vi "R45.vi"() -> ()   [LabVIEW 2016, in "beamline sections.lvlib"]
uses:
  controls/beamline sections.lvlib
  save load/saveloadprev.ctl
  <vilib>/Instr/_visa.llb/VISA Open Access Mode.ctl
  sub-VIs/sub-VIs.lvlib
  save load/SaveLoad.lvlib
panel:
  in  "Tab Control":T1(tab)
  out "ExB 2":bool
  in  "GFM Field set":dbl(slide) min=0.0 max=150.0 scale=0.0..2.0
  in  "ExB #2 Electric":dbl(slide) min=0.0 max=200.0 scale=0.0..60.0
  in  "Reset ExB 2":bool
  in  "ExB #1 Electric":dbl(slide) min=0.0 max=200.0 scale=0.0..60.0
  out "R45 Steerer Y Read":dbl format="%#.2g"
  out "R45 Steerer X Read":dbl format="%#.2g"
  in  "R45 Y steerer":dbl(slide) min=-10.0 max=10.0 scale=-10.0..10.0
  in  "R45 Quad A":dbl(slide) min=0.0 max=200.0 scale=0.0..120.0
  in  "R45 X steerer":dbl(slide) min=-10.0 max=10.0 scale=-10.0..10.0
  out "R45 Steerer":bool
  out "R45 quad Range":bool
  in  "R45 Quad B":dbl(slide) min=0.0 max=200.0 scale=0.0..120.0
  in  "stop":bool
  out "ExB 1":bool
  out "ExB 1- V":dbl format="%#.2g"
  in  "ExB #1 Magnet":dbl(slide) scale=0.0..30.0
  out "ExB 1+ V":dbl format="%#.2g"
  out "read current quad B":string
  out "read voltage quad B":string
  out "read current quad A":string
  out "read voltage Quad A":string
  in  "ExB #2 Magnet":dbl(slide) scale=0.0..30.0
  in  "Preview-Save-Load":T2
  out "ExB 2+ I":dbl
  out "ExB 2- I":dbl
  out "ExB 2- V":dbl
  out "ExB 2+ V":dbl
  out "ExB 1+ I":dbl
  out "ExB 1- I":dbl
  out "GFM field read":dbl
  out "Left-Steerer V read":dbl
  out "Down-Steerer V read":dbl
  out "Up-Steerer V read":dbl
  out "Right-Steerer V read":dbl
  out "Left-Steerer I read":dbl
  out "Right-Steerer I read":dbl
  out "Down-Steerer I read":dbl
  out "Up-Steerer I read":dbl
  in  "R45 temp file":path=path "D:/Main Tune Parameters/Temp Configs/R45.txt"
  in  "Quad A VISA GPIB Resource":refnum<visa-resource-name>="GPIB1::6::INSTR"
  in  "Quad B VISA GPIB Resource":refnum<visa-resource-name>="GPIB1::3::INSTR"
  out "SV error":errorcluster
  out "Quad B error":errorcluster
  out "Quad A error":errorcluster
  out "GFM SV error":errorcluster
  out "SaveLoad error":errorcluster
  out "R45-2-RT Error":errorcluster
  out "R45-2-FPGA Error":errorcluster
  out "R45-1-RT Error":errorcluster
  out "R45-1-FPGA Error":errorcluster
  # "R45"
  # "R45 X and Y steerers are split between Up/Down (Y) and Right/Left (X)"
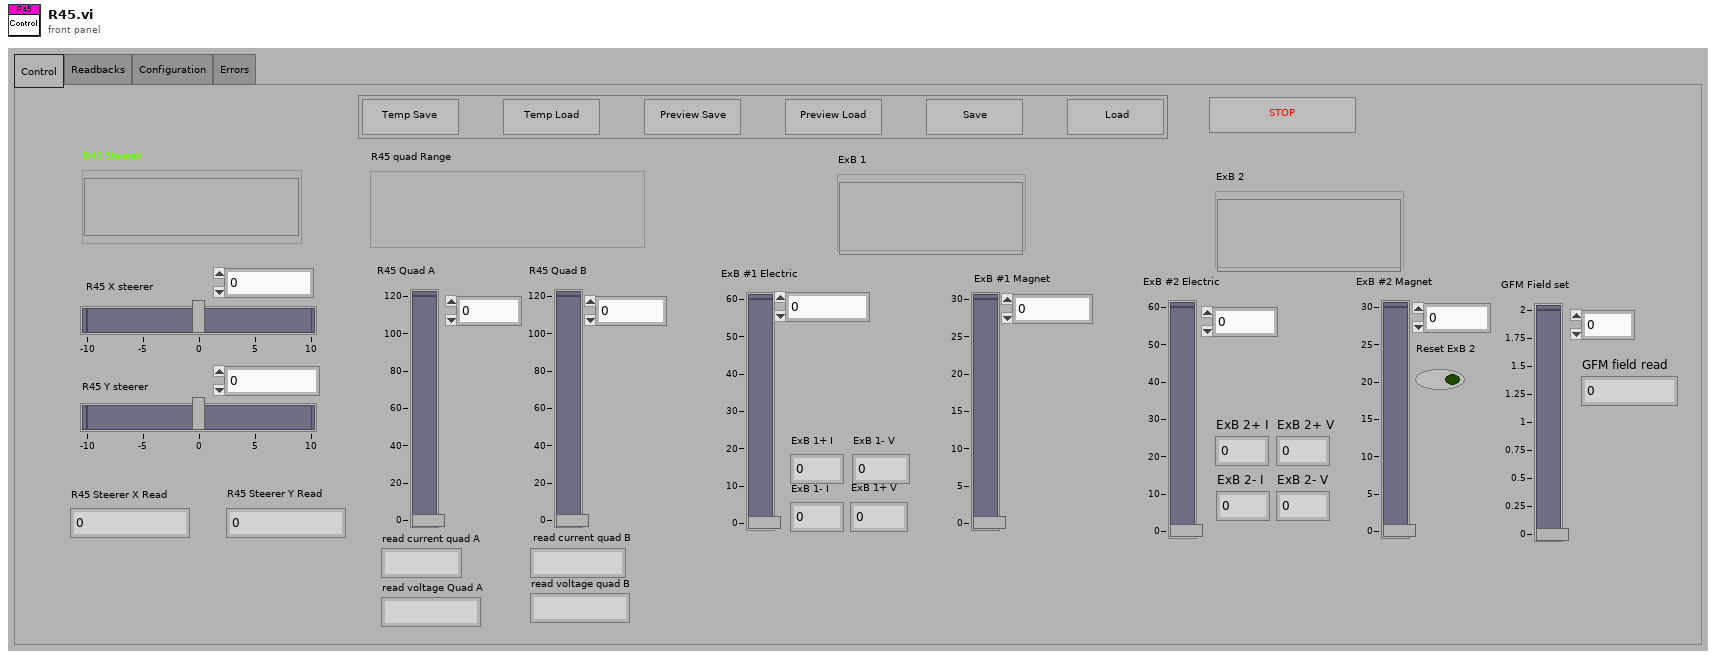
[diagram p1: front panel]
types:
  T1 = enum32{"Control", "Readbacks", "Configuration", "Errors"}
  T2 = typedef "saveloadprev.ctl" = cluster{"Temp Save":bool, "Temp Load":bool, "Save":bool, "Load":bool, "Preview Save":bool, "Preview Load":bool}
  T3 = typedef "VISA Open Access Mode.ctl" = u32
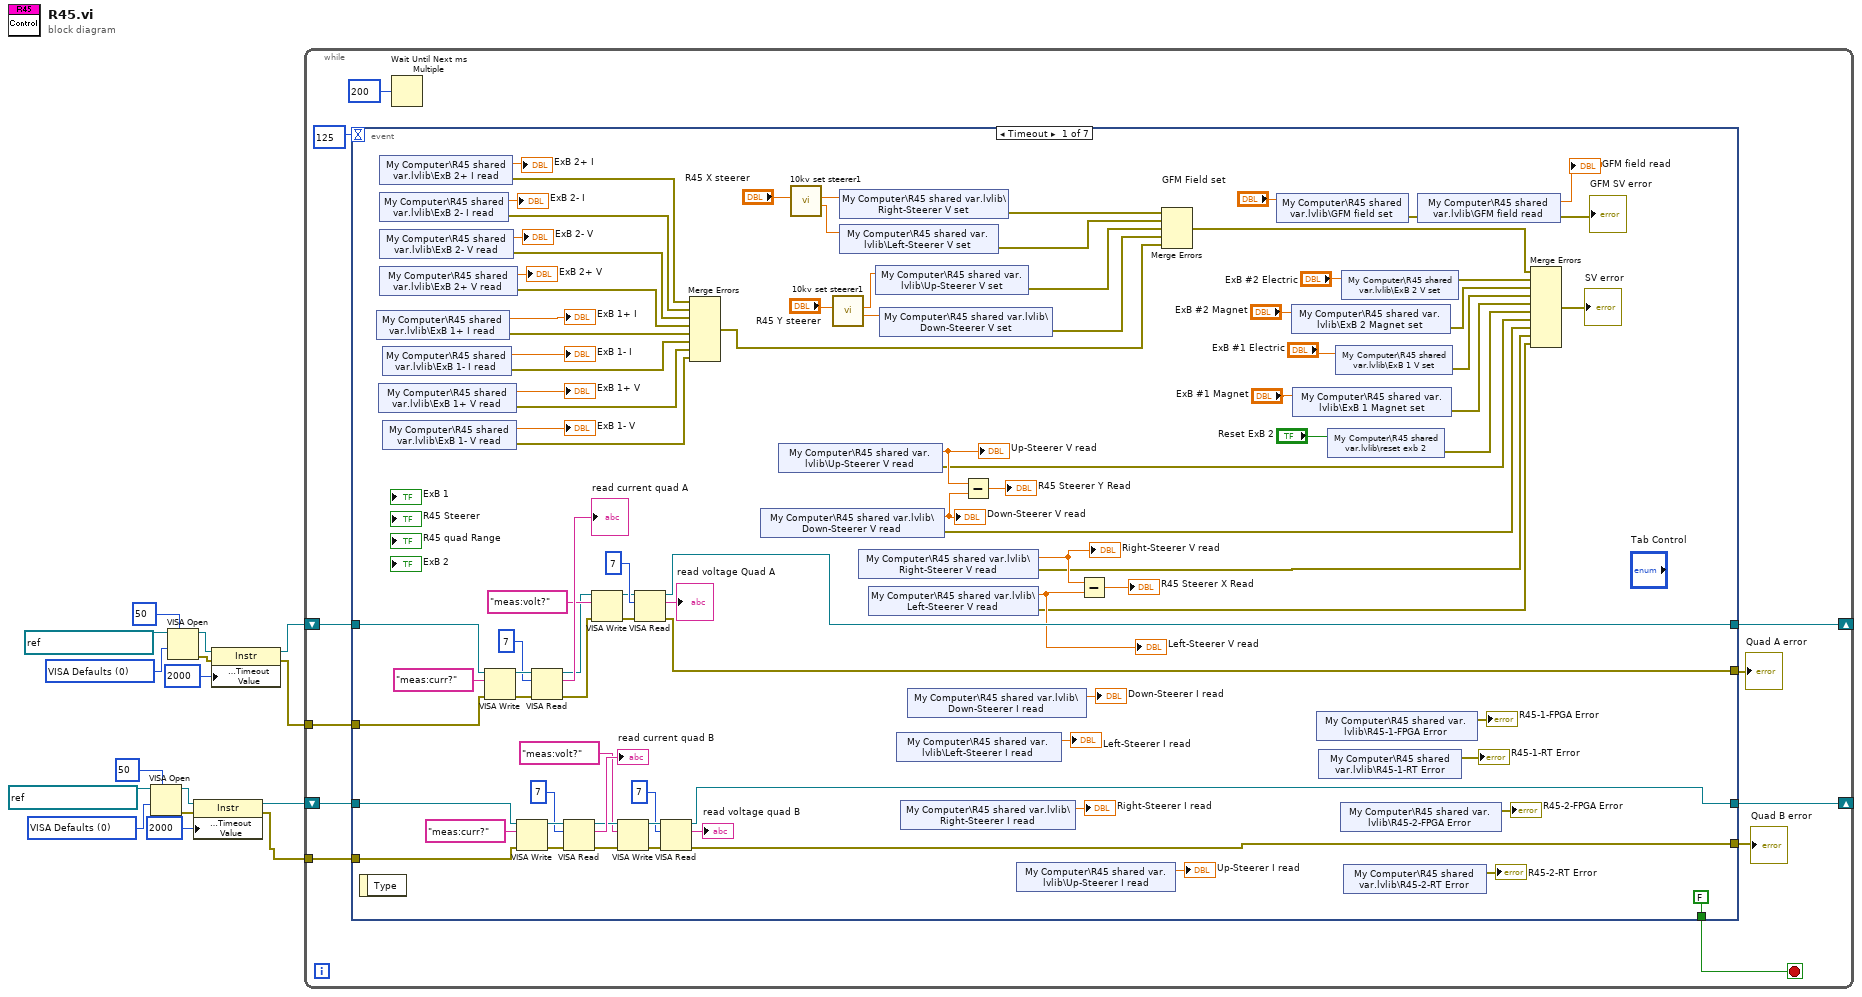
[diagram p0: block diagram]
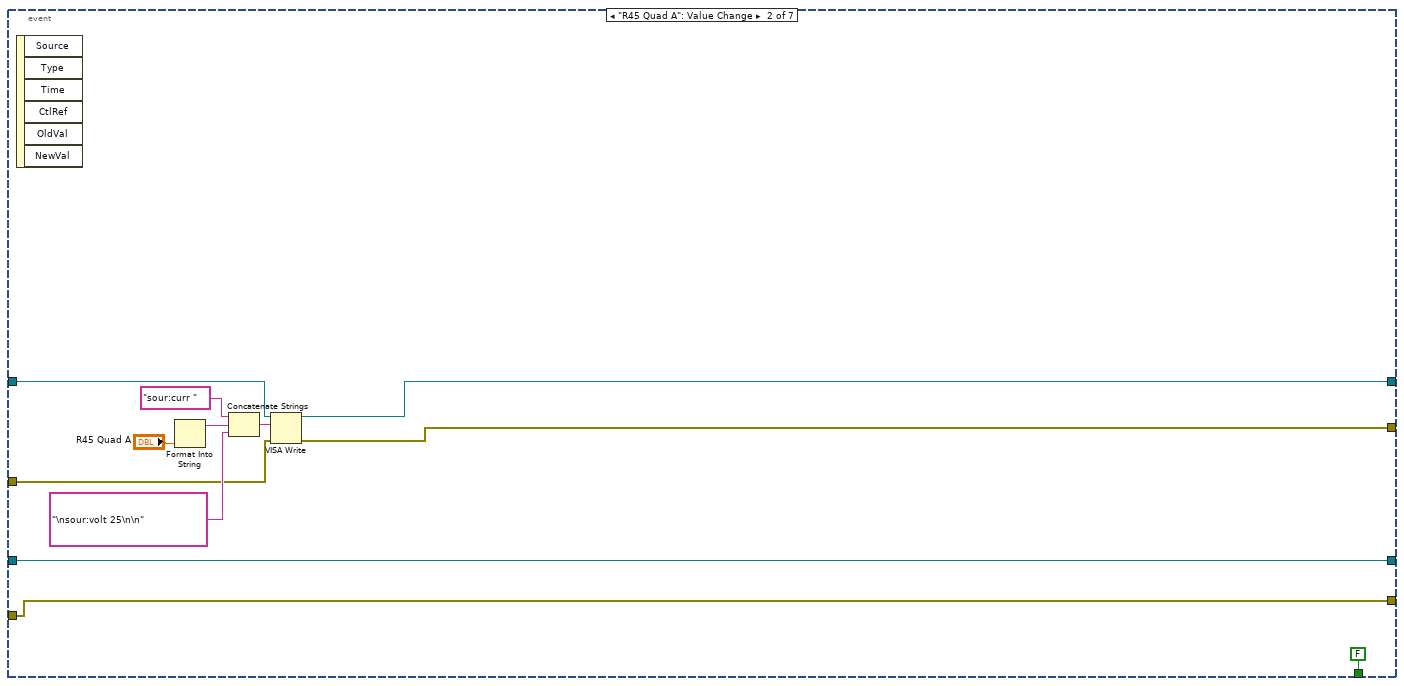
[diagram p2: hidden frame]
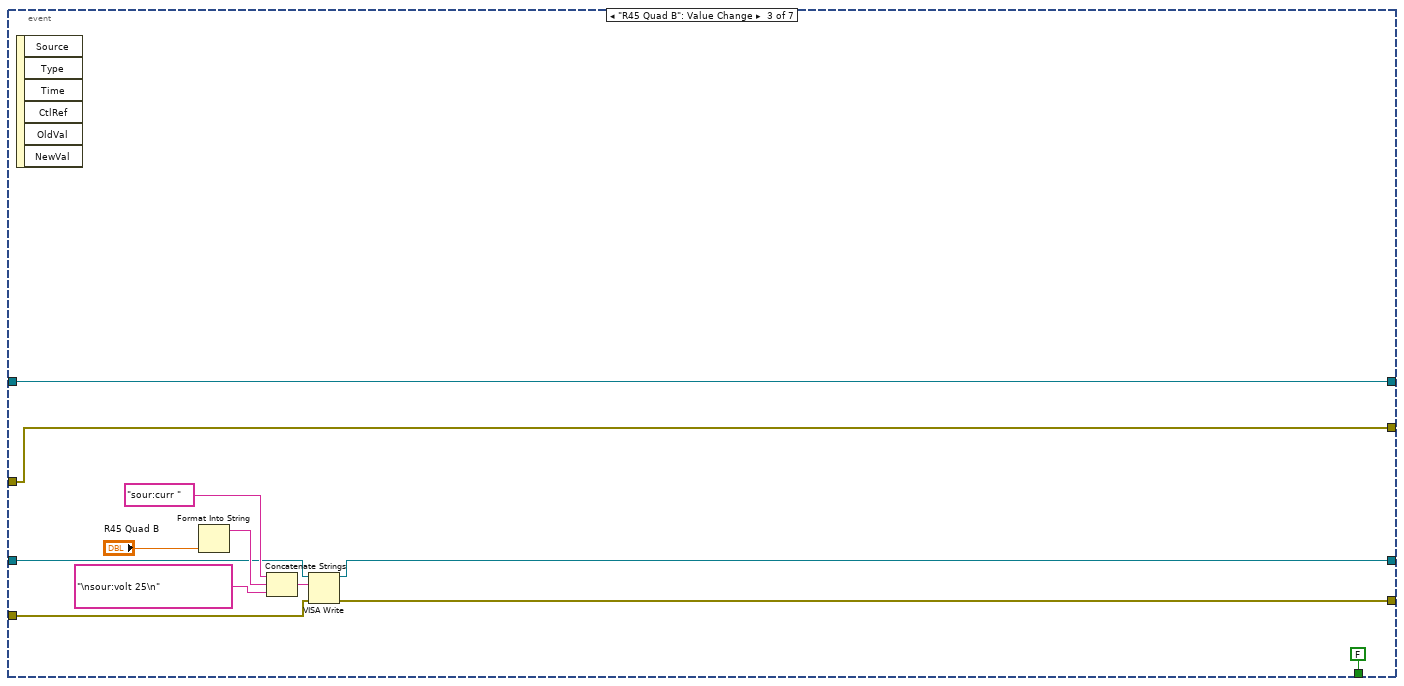
[diagram p3: hidden frame]
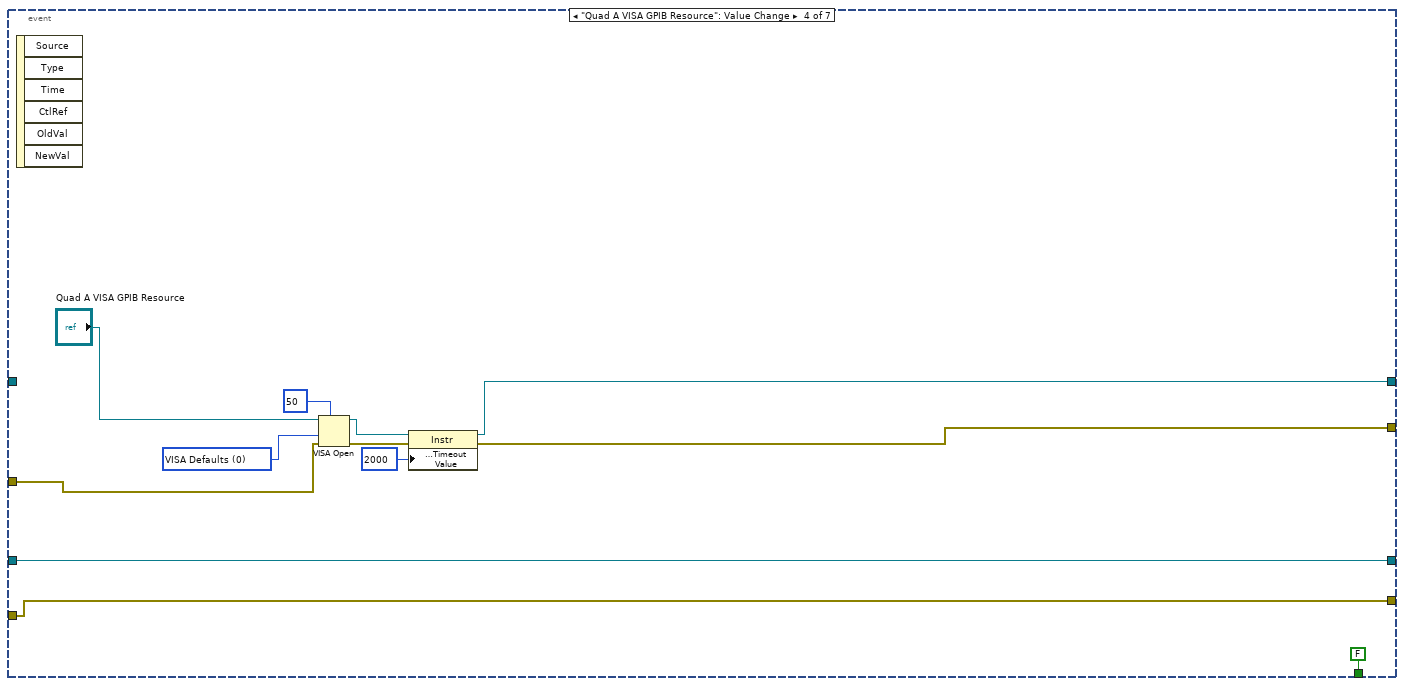
[diagram p4: hidden frame]
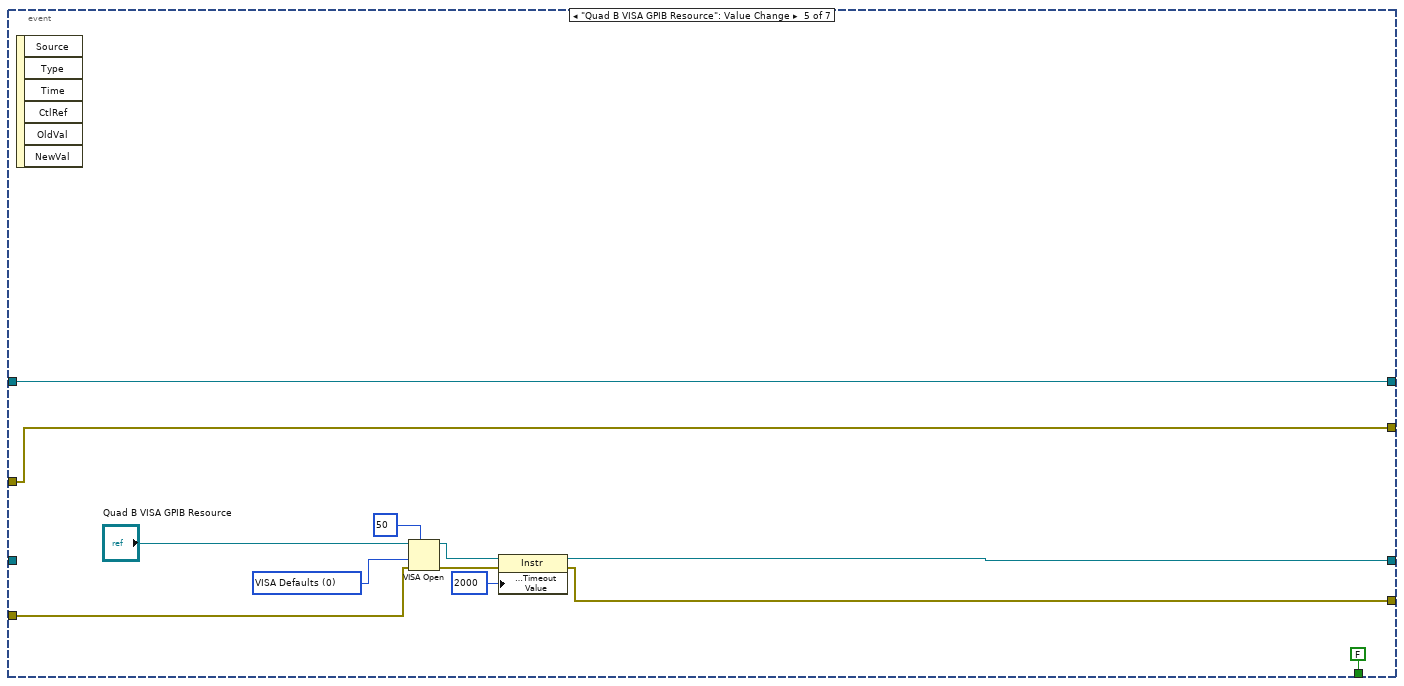
[diagram p5: hidden frame]
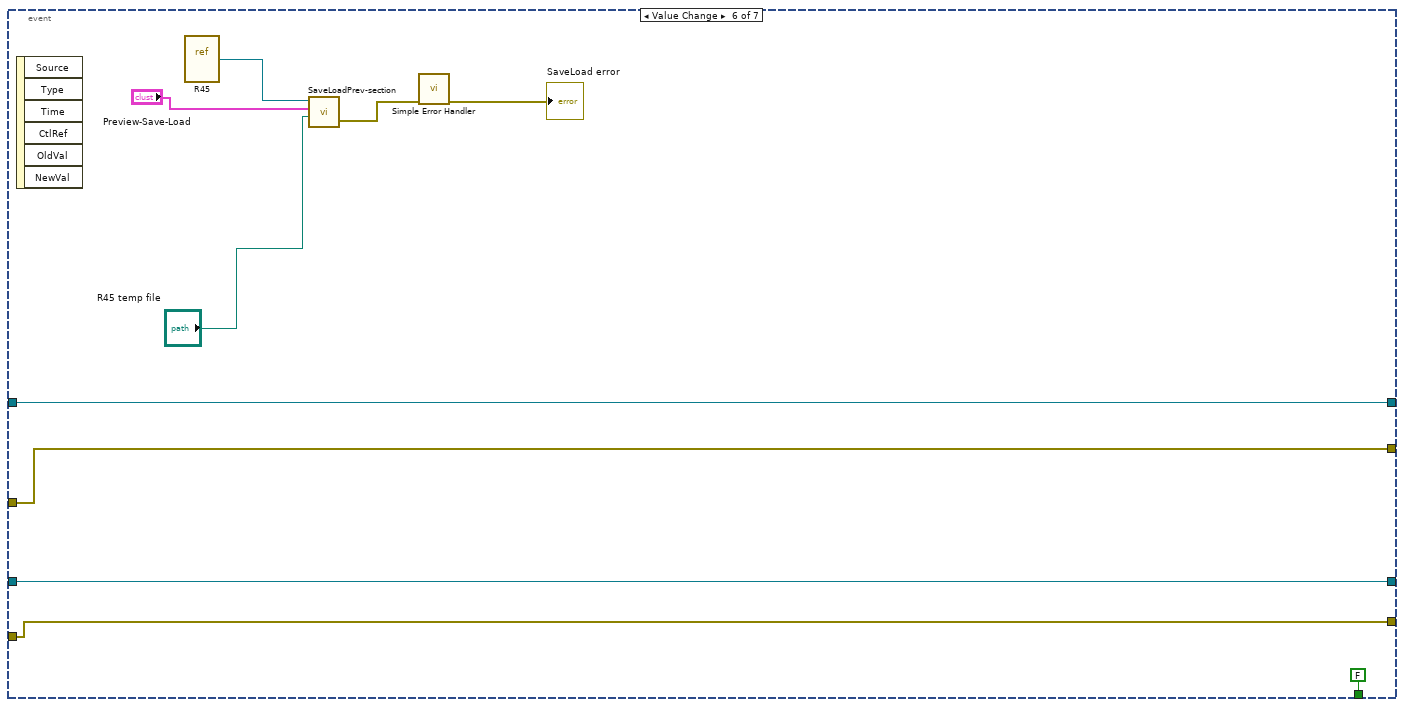
[diagram p6: hidden frame]
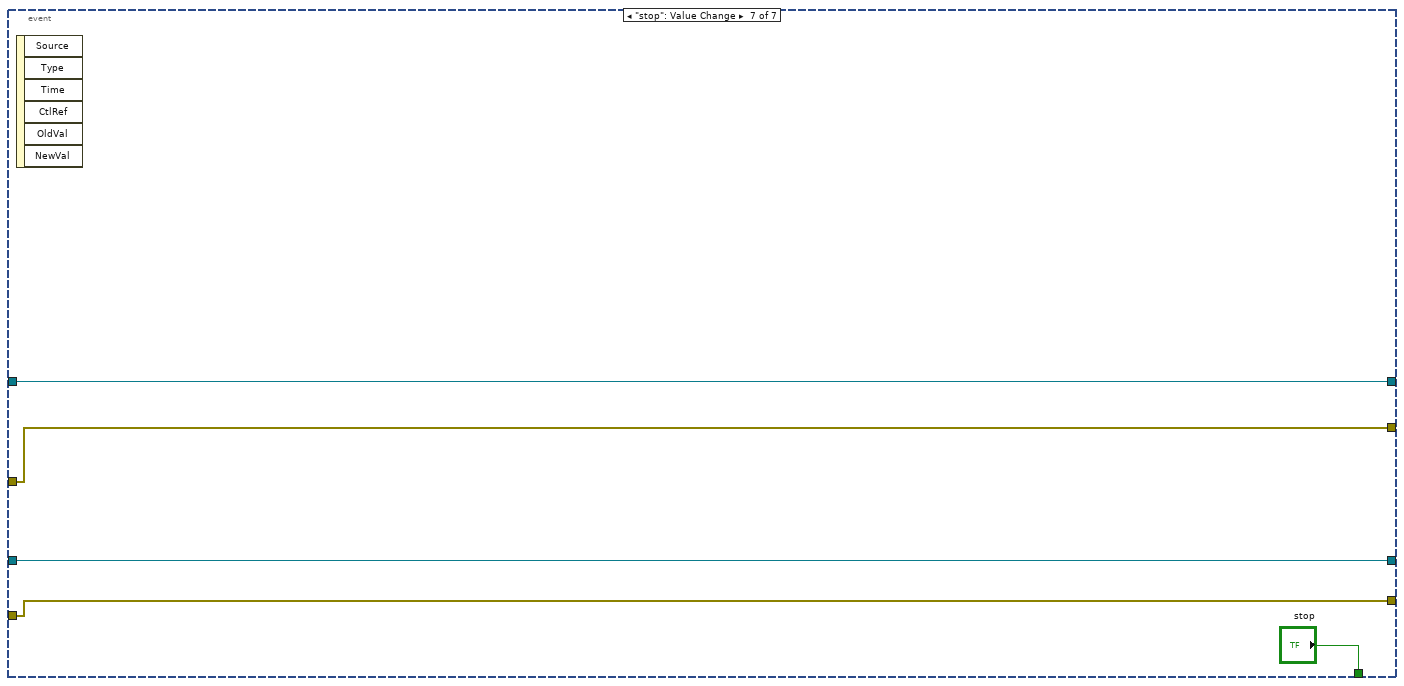
[diagram p7: hidden frame]
diagram:
  w15 = T3 0 items=["VISA Defaults"=0, "Exclusive Lock"=1, "Load Configured Settings"=4] ("Access Mode")
  w6 = T3 0 items=["VISA Defaults"=0, "Exclusive Lock"=1, "Load Configured Settings"=4] ("Access Mode")
  n1 = VISA Open(timeout (0)=u32 50 ("VISA Open timeout (0)"), access mode=w6, VISA resource name=refnum<visa-resource-name> "GPIB1::6::INSTR" ("VISA GPIB Resource")) -> (VISA resource name=w10:refnum<visa-resource-name>, error out=w11:errorcluster)  [unwired: 2 in]
  n2 = VISA Open(timeout (0)=u32 50 ("VISA Open timeout (0)"), access mode=w15, VISA resource name=refnum<visa-resource-name> "GPIB1::3::INSTR" ("VISA GPIB Resource")) -> (VISA resource name=w1:refnum<visa-resource-name>, error out=w12:errorcluster)  [unwired: 2 in]
  n3 = property class="Instr"(reference=w10, error in=w11, "General Settings:Timeout Value"=u32 2000) -> (reference out=w2:refnum<visa-resource-name>, error out=w3:errorcluster)
  n4 = property class="Instr"(reference=w1, error in=w12, "General Settings:Timeout Value"=u32 2000) -> (reference out=w5:refnum<visa-resource-name>, error out=w4:errorcluster)
  n5 = while {
    tunnel: w4 -> [w25]
    tunnel: w3 -> [w23]
    shift-right: [w20] -> _
    shift-left: w2 -> [w22]
    shift-right: [w19] -> _
    shift-left: w5 -> [w26]
    stop <- w27 stop-if-true
    n6 = event shown="[0] Timeout" {
      selector: _ -> [_ _ _ _ _ _ _]
      dyn-events: _ -> [_ _ _ _ _ _ _]
      timeout: 125 -> [_ _ _ _ _ _ _]
      tunnel: [FALSE ("stop") FALSE ("stop") FALSE ("stop") FALSE ("stop") FALSE ("stop") FALSE ("stop") "stop"] -> w27
      tunnel: w26 -> [w92 w127 w134 _ w158 w178 w180]
      tunnel: w25 -> [w93 w126 w135 w151 w159 w177 w181]
      tunnel: [w91 w124 w135 w148 w159 w177 w181] -> w24
      tunnel: w23 -> [w107 w122 w139 w146 w163 w175 w182]
      tunnel: w22 -> [w108 w123 w138 w147 _ w176 w183]
      tunnel: [w106 w122 w137 w146 w160 w175 w182] -> w21
      tunnel: [w65 w123 w136 w147 w161 w176 w183] -> w20
      tunnel: [w90 w125 w134 w149 w158 w178 w180] -> w19
      event Timeout {
        n7 = event-data() -> ()  [unwired: 1 in, 1 out]
        n8 = shared-variable "My Computer\\R45 shared var.lvlib\\ExB 1+ I read"() -> (→"ExB 1+ I":dbl, error out=w70:errorcluster)  [unwired: 1 in]
        n9 = shared-variable "My Computer\\R45 shared var.lvlib\\ExB 1+ V read"() -> (→"ExB 1+ V":dbl, error out=w68:errorcluster)  [unwired: 1 in]
        n10 = shared-variable "My Computer\\R45 shared var.lvlib\\ExB 2+ I read"() -> (→"ExB 2+ I":dbl, error out=w33:errorcluster)  [unwired: 1 in]
        n11 = shared-variable "My Computer\\R45 shared var.lvlib\\ExB 2- I read"() -> (→"ExB 2- I":dbl, error out=w34:errorcluster)  [unwired: 1 in]
        n12 = shared-variable "My Computer\\R45 shared var.lvlib\\ExB 2- V read"() -> (→"ExB 2- V":dbl, error out=w35:errorcluster)  [unwired: 1 in]
        n13 = shared-variable "My Computer\\R45 shared var.lvlib\\ExB 2+ V read"() -> (→"ExB 2+ V":dbl, error out=w36:errorcluster)  [unwired: 1 in]
        n14 = shared-variable "My Computer\\R45 shared var.lvlib\\ExB 1- I read"() -> (→"ExB 1- I":dbl, error out=w69:errorcluster)  [unwired: 1 in]
        n15 = shared-variable "My Computer\\R45 shared var.lvlib\\ExB 1- V read"() -> (→"ExB 1- V":dbl, error out=w67:errorcluster)  [unwired: 1 in]
        n16 = VISA Write(VISA resource name=w92, write buffer="meas:curr?" ("string"), error in (no error)=w93) -> (VISA resource name out=w104:refnum<visa-resource-name>, error out=w94:errorcluster)  [unwired: 1 out]
        n17 = VISA Write(VISA resource name=w108, write buffer="meas:curr?" ("string"), error in (no error)=w107) -> (VISA resource name out=w119:refnum<visa-resource-name>, error out=w120:errorcluster)  [unwired: 1 out]
        n18 = VISA Read(VISA resource name=w104, byte count=u32 7, error in (no error)=w94) -> (VISA resource name out=w99:refnum<visa-resource-name>, read buffer=→"read current quad A":string, error out=w95:errorcluster)  [unwired: 1 out]
        n19 = VISA Read(VISA resource name=w119, byte count=u32 7, error in (no error)=w120) -> (VISA resource name out=w112:refnum<visa-resource-name>, read buffer=→"read current quad B":string, error out=w111:errorcluster)  [unwired: 1 out]
        n20 = VISA Write(VISA resource name=w99, write buffer="meas:volt?", error in (no error)=w95) -> (VISA resource name out=w97:refnum<visa-resource-name>, error out=w101:errorcluster)  [unwired: 1 out]
        n21 = VISA Write(VISA resource name=w112, write buffer="meas:volt?", error in (no error)=w111) -> (VISA resource name out=w114:refnum<visa-resource-name>, error out=w109:errorcluster)  [unwired: 1 out]
        n22 = VISA Read(VISA resource name=w97, byte count=u32 7, error in (no error)=w101) -> (VISA resource name out=w90:refnum<visa-resource-name>, read buffer=→"read voltage Quad A":string, error out=w91:errorcluster)  [unwired: 1 out]
        n23 = VISA Read(VISA resource name=w114, byte count=u32 7, error in (no error)=w109) -> (VISA resource name out=w65:refnum<visa-resource-name>, read buffer=→"read voltage quad B":string, error out=w106:errorcluster)  [unwired: 1 out]
        n24 = Merge Errors(w33, w34, w35, w36, w70, w69, w68, w67) -> (w32:errorcluster)
        n25 = shared-variable "My Computer\\R45 shared var.lvlib\\Down-Steerer V read"() -> (w49:dbl, error out=w47:errorcluster)  [unwired: 1 in]
        "Down-Steerer V read" <- w49
        n26 = shared-variable "My Computer\\R45 shared var.lvlib\\Up-Steerer V read"() -> (w50:dbl, error out=w46:errorcluster)  [unwired: 1 in]
        "Up-Steerer V read" <- w50
        n27 = call "10kv set steerer1.vi"("Steerer Control IN"="R45 X steerer") -> ("- Steerer"=w61:dbl, "+ Steerer"=w62:dbl)  [unwired: 8 in, 1 out]
        n28 = call "10kv set steerer1.vi"("Steerer Control IN"="R45 Y steerer") -> ("- Steerer"=w59:dbl, "+ Steerer"=w60:dbl)  [unwired: 8 in, 1 out]
        n29 = shared-variable "My Computer\\R45 shared var.lvlib\\Right-Steerer V set"(w62) -> (error out=w55:errorcluster)  [unwired: 1 in]
        n30 = shared-variable "My Computer\\R45 shared var.lvlib\\Left-Steerer V set"(w61) -> (error out=w56:errorcluster)  [unwired: 1 in]
        n31 = shared-variable "My Computer\\R45 shared var.lvlib\\Right-Steerer V read"() -> (w45:dbl, error out=w41:errorcluster)  [unwired: 1 in]
        "Right-Steerer V read" <- w45
        n32 = shared-variable "My Computer\\R45 shared var.lvlib\\Left-Steerer V read"() -> (w44:dbl, error out=w42:errorcluster)  [unwired: 1 in]
        "Left-Steerer V read" <- w44
        n33 = shared-variable "My Computer\\R45 shared var.lvlib\\Up-Steerer V set"(w60) -> (error out=w57:errorcluster)  [unwired: 1 in]
        n34 = shared-variable "My Computer\\R45 shared var.lvlib\\Down-Steerer V set"(w59) -> (error out=w58:errorcluster)  [unwired: 1 in]
        n35 = shared-variable "My Computer\\R45 shared var.lvlib\\Left-Steerer I read"() -> (→"Left-Steerer I read":dbl)  [unwired: 1 in, 1 out]
        n36 = shared-variable "My Computer\\R45 shared var.lvlib\\Right-Steerer I read"() -> (→"Right-Steerer I read":dbl)  [unwired: 1 in, 1 out]
        n37 = shared-variable "My Computer\\R45 shared var.lvlib\\Down-Steerer I read"() -> (→"Down-Steerer I read":dbl)  [unwired: 1 in, 1 out]
        n38 = Subtract(x=w50, y=w49) -> (x-y=→"R45 Steerer Y Read":dbl)
        n39 = shared-variable "My Computer\\R45 shared var.lvlib\\Up-Steerer I read"() -> (→"Up-Steerer I read":dbl)  [unwired: 1 in, 1 out]
        n40 = Subtract(x=w45, y=w44) -> (x-y=→"R45 Steerer X Read":dbl)
        n41 = Merge Errors(w55, w56, w57, w58, w32) -> (w66:errorcluster)
        n42 = shared-variable "My Computer\\R45 shared var.lvlib\\GFM field set"("GFM Field set") -> (error out=w88:errorcluster)  [unwired: 1 in]
        n43 = shared-variable "My Computer\\R45 shared var.lvlib\\ExB 2 Magnet set"("ExB #2 Magnet") -> (error out=w72:errorcluster)  [unwired: 1 in]
        n44 = shared-variable "My Computer\\R45 shared var.lvlib\\ExB 1 Magnet set"("ExB #1 Magnet") -> (error out=w74:errorcluster)  [unwired: 1 in]
        n45 = shared-variable "My Computer\\R45 shared var.lvlib\\R45-1-FPGA Error"() -> (→"R45-1-FPGA Error":errorcluster)  [unwired: 1 in, 1 out]
        n46 = shared-variable "My Computer\\R45 shared var.lvlib\\R45-1-RT Error"() -> (→"R45-1-RT Error":errorcluster)  [unwired: 1 in, 1 out]
        n47 = shared-variable "My Computer\\R45 shared var.lvlib\\reset exb 2"("Reset ExB 2") -> (error out=w75:errorcluster)  [unwired: 1 in]
        n48 = shared-variable "My Computer\\R45 shared var.lvlib\\ExB 1 V set"("ExB #1 Electric") -> (error out=w73:errorcluster)  [unwired: 1 in]
        n49 = shared-variable "My Computer\\R45 shared var.lvlib\\R45-2-FPGA Error"() -> (→"R45-2-FPGA Error":errorcluster)  [unwired: 1 in, 1 out]
        n50 = shared-variable "My Computer\\R45 shared var.lvlib\\ExB 2 V set"("ExB #2 Electric") -> (error out=w71:errorcluster)  [unwired: 1 in]
        n51 = shared-variable "My Computer\\R45 shared var.lvlib\\R45-2-RT Error"() -> (→"R45-2-RT Error":errorcluster)  [unwired: 1 in, 1 out]
        n52 = shared-variable "My Computer\\R45 shared var.lvlib\\GFM field read"(error in=w88) -> (→"GFM field read":dbl, error out=→"GFM SV error":errorcluster)
        n53 = Merge Errors(w66, w71, w72, w73, w74, w75, w46, w47, w41, w42) -> (→"SV error":errorcluster)
      }
      event "R45 Quad A": Value Change {
        n54 = event-data() -> ()  [unwired: 1 in, 6 out]
        n55 = Format Into String("R45 Quad A") -> (resulting string=w128:string)  [unwired: 3 in, 1 out]
        n56 = Concatenate Strings("sour:curr " ("string"), w128, "\nsour:volt 25\n\n" ("write buffer")) -> (w129:string)
        n57 = VISA Write(VISA resource name=w127, write buffer=w129, error in (no error)=w126) -> (VISA resource name out=w125:refnum<visa-resource-name>, error out=w124:errorcluster)  [unwired: 1 out]
      }
      event "R45 Quad B": Value Change {
        n58 = event-data() -> ()  [unwired: 1 in, 6 out]
        n59 = Format Into String("R45 Quad B") -> (resulting string=w140:string)  [unwired: 3 in, 1 out]
        n60 = Concatenate Strings("sour:curr " ("string"), w140, "\nsour:volt 25\n" ("write buffer")) -> (w142:string)
        n61 = VISA Write(VISA resource name=w138, write buffer=w142, error in (no error)=w139) -> (VISA resource name out=w136:refnum<visa-resource-name>, error out=w137:errorcluster)  [unwired: 1 out]
      }
      event "Quad A VISA GPIB Resource": Value Change {
        w155 = T3 0 items=["VISA Defaults"=0, "Exclusive Lock"=1, "Load Configured Settings"=4] ("Access Mode")
        n62 = event-data() -> ()  [unwired: 1 in, 6 out]
        n63 = VISA Open(timeout (0)=u32 50 ("VISA Open timeout (0)"), access mode=w155, error in (no error)=w151, VISA resource name="Quad A VISA GPIB Resource") -> (VISA resource name=w153:refnum<visa-resource-name>, error out=w152:errorcluster)  [unwired: 1 in]
        n64 = property class="Instr"(reference=w153, error in=w152, "General Settings:Timeout Value"=u32 2000) -> (reference out=w149:refnum<visa-resource-name>, error out=w148:errorcluster)
      }
      event "Quad B VISA GPIB Resource": Value Change {
        w167 = T3 0 items=["VISA Defaults"=0, "Exclusive Lock"=1, "Load Configured Settings"=4] ("Access Mode")
        n65 = event-data() -> ()  [unwired: 1 in, 6 out]
        n66 = VISA Open(timeout (0)=u32 50 ("VISA Open timeout (0)"), access mode=w167, error in (no error)=w163, VISA resource name="Quad B VISA GPIB Resource") -> (VISA resource name=w165:refnum<visa-resource-name>, error out=w164:errorcluster)  [unwired: 1 in]
        n67 = property class="Instr"(reference=w165, error in=w164, "General Settings:Timeout Value"=u32 2000) -> (reference out=w161:refnum<visa-resource-name>, error out=w160:errorcluster)
      }
      event Value Change {
        n68 = event-data() -> ()  [unwired: 1 in, 6 out]
        n69 = vi-ref "R45.vi"() -> (w173:refnum<vi>)
        n70 = call "SaveLoadPrev-section.vi"("file path (use dialog)"="R45 temp file", "Cluster 2"="Preview-Save-Load", "VI Refnum"=w173) -> ("error out"=w171:errorcluster)  [unwired: 2 in]
        n71 = call <vilib>:"Simple Error Handler.vi"("error in (no error)"=w171) -> ("error out"=→"SaveLoad error":errorcluster)  [unwired: 4 in, 4 out]
      }
      event "stop": Value Change {
        n72 = event-data() -> ()  [unwired: 1 in, 6 out]
      }
    }
    "Quad A error" <- w24
    "Quad B error" <- w21
    n73 = Wait Until Next ms Multiple(millisecond multiple=u32 200) -> ()  [unwired: 1 out]
  }
